vi "GetMethods.vi"(0 "ClassReaderNative in":refnum<class "ClassReaderNative.lvclass">, 5 "error in (no error)":errorcluster) -> (14 "ClassReaderNative out":refnum<class "ClassReaderNative.lvclass">, 15 "Methods":T1[](array[typedef]), 16 "Constructor/CreateIndex":i32, 19 "error out":errorcluster)   [LabVIEW 2014, in "ClassReaderNative.lvclass"]
uses:
  <resource>/Framework/Providers/Open_GDS/ClassProviders/Provider_LvNativeClass/ClassReaderNative_class/ClassReaderNative.lvclass
  <resource>/Framework/Providers/Open_GDS/ClassProviders/Provider_BaseClassInterface/Types/ClassTypes_MethodType.ctl
  <resource>/Framework/Providers/Open_GDS/ClassProviders/Provider_LvNativeClass/ClassReaderNative_class/ClassReaderNative.lvclass/ClassReaderNative.ctl
  <resource>/Framework/Providers/Open_GDS/ClassProviders/Provider_BaseClassInterface/ClassReader_class/ClassReader.lvclass
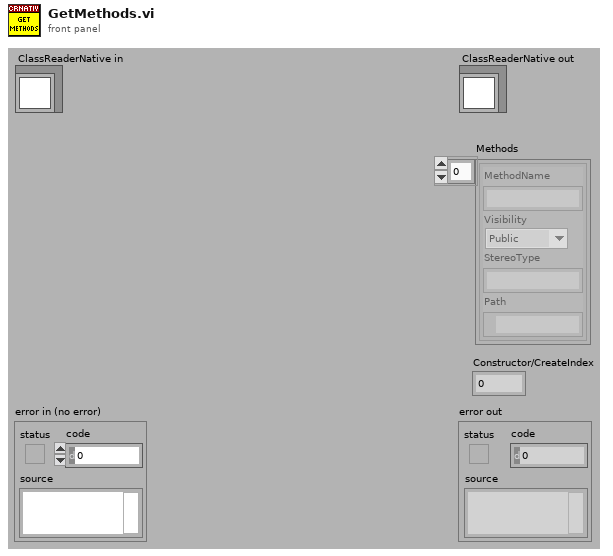
[diagram p1: front panel]
types:
  T1 = typedef "ClassTypes_MethodType.ctl" = cluster{"MethodName":string, "Visibility":enum16{"Public", "Private", "Protected"}, "StereoType":string, "Path":path}
  T2 = enum32{"invalid VI type", "Standard VI", "Control VI", "Global VI", "Polymorphic VI", "Configuration VI", "SubSystem", "Facade VI", "Method VI", "Statechart Diagram VI"}
  T3 = enum32{"invalid scope", "public", "private", "protected", "community"}
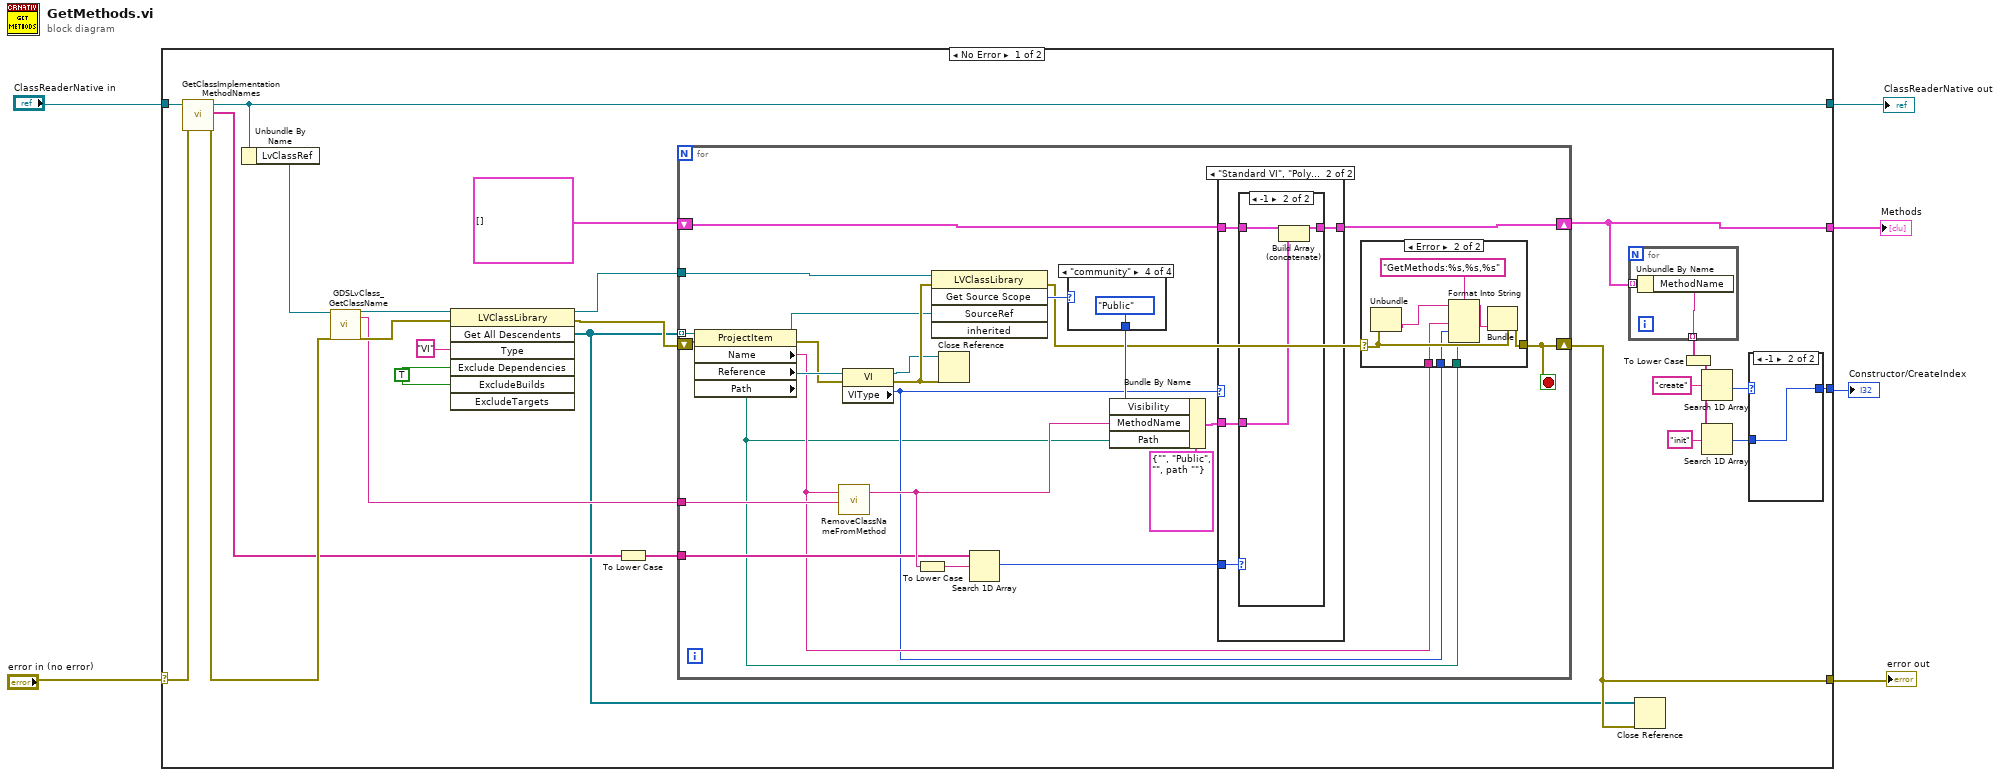
[diagram p0: block diagram]
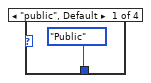
[diagram p6: hidden frame]
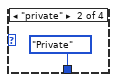
[diagram p7: hidden frame]
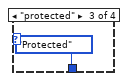
[diagram p8: hidden frame]
diagram:
  n1 = case shown="No Error" "error in (no error)" {
    selector: "error in (no error)" -> [w13 w82]
    tunnel: "ClassReaderNative in" -> [w15 w83]
    tunnel: [w14 w83] -> w4
    tunnel: [w23 _] -> w3
    tunnel: [w8 w82] -> w2
    tunnel: [w17 _] -> w1
    frame No Error {
      w9 = TRUE ("ExcludeDependencies")
      n2 = call-dynamic "GetClassImplementationMethodNames.vi"("error in (no error)"=w13, "ClassReaderNative in"=w15) -> ("error out"=w12:errorcluster, "ImplementationMethodNames"=w11:string[], "ClassReaderNative out"=w14:refnum<class "ClassReaderNative.lvclass">)  [unwired: 7 in]
      n3 = Unbundle By Name(w14) -> ("LvClassRef"=w24:refnum<vi>)
      n4 = call <resource>:"GDSLvClass_GetClassName.vi"("ViRef/Path,LvClassRef/Path"=w24, "error in (no error)"=w12) -> ("ClassRef"=w27:refnum<vi>, "ClassName(without .lvclass)"=w25:string, "error out"=w26:errorcluster)  [unwired: 15 in]
      n5 = invoke class="LVClassLibrary" method="Get All Descendents"(reference=w27, error in=w26, "Type"="VI", "Exclude Dependencies"=w9, "ExcludeBuilds"=w9) -> (reference out=w30:refnum<vi>, error out=w29:errorcluster, "All Descendents"=w7:refnum<vi>[])  [unwired: 2 in, 4 out]
      n6 = To Lower Case(string=w11) -> (all lower case string=w10:string[])
      n7 = for {
        tunnel: w7 -> [w59] mode=indexing
        tunnel: w30 -> [w58]
        shift-right: [w39] -> w8
        shift-left: w29 -> [w56]
        shift-right: [w53] -> w23
        shift-left: T1[] [] ("Methods") -> [w54]
        tunnel: w25 -> [w46]
        tunnel: w10 -> [w43]
        stop <- w39 stop-if-true
        n8 = property class="ProjectItem"(reference=w59, error in=w56) -> (reference out=w47:refnum<vi>, error out=w50:errorcluster, "Name"=w38:string, "Reference"=w55:refnum<vi>, "Path"=w36:path)
        n9 = call <resource>:"RemoveClassNameFromMethod.vi"("MethodVINameIn"=w38, "ClassName"=w46) -> ("MethodVINameOut"=w44:string)  [unwired: 17 in]
        n10 = property class="VI"(reference=w55, error in=w50) -> (reference out=w48:refnum<vi>, error out=w49:errorcluster, "VIType"=w37:T2)
        n11 = To Lower Case(string=w44) -> (all lower case string=w42:string)
        n12 = invoke class="LVClassLibrary" method="Get Source Scope"(reference=w58, error in=w49, "SourceRef"=w47) -> (error out=w40:errorcluster, "GetSourceScope"=w57:T3)  [unwired: 2 in, 3 out]
        n13 = Close Reference(reference=w48, error in (no error)=w49) -> ()  [unwired: 1 out]
        n14 = Search 1D Array(1D array=w43, element=w42) -> (index of element=w45:i32)  [unwired: 1 in]
        n15 = case shown="\"community\"" w57 {
          tunnel: [enum16{"Public", "Private", "Protected"}."Public" ("Visibility") enum16{"Public", "Private", "Protected"}."Private" ("Visibility") enum16{"Public", "Private", "Protected"}."Protected" ("Visibility") enum16{"Public", "Private", "Protected"}."Public" ("Visibility")] -> w41
          frame "public", Default {
          }
          frame "private" {
          }
          frame "protected" {
          }
          frame "community" {
          }
        }
        n16 = Bundle By Name(cluster=T1 {"MethodName"="", "Visibility"=enum."Public", "StereoType"="", "Path"=path ""} ("Method"), "Visibility"=w41, "MethodName"=w44, "Path"=w36) -> (w51:T1)
        n17 = case shown="\"Standard VI\", \"Polymorphic VI\", \"Facade VI\", \"Method VI\"" w37 {
          tunnel: w54 -> [w69 w73]
          tunnel: [w69 w72] -> w53
          tunnel: w51 -> [_ w71]
          tunnel: w45 -> [_ w70]
          frame Default {
          }
          frame "Standard VI", "Polymorphic VI", "Facade VI", "Method VI" {
            n18 = case shown="-1" w70 {
              tunnel: w73 -> [w74 w77]
              tunnel: [w74 w76] -> w72
              tunnel: w71 -> [_ w75]
              frame 0, Default {
              }
              frame -1 {
                n19 = Build Array (concatenate)(w77, w75) -> (w76:T1[])
              }
            }
          }
        }
        n20 = case shown="Error" w40 {
          selector: w40 -> [w60 w68]
          tunnel: [w60 w67] -> w39
          tunnel: w38 -> [_ w63]
          tunnel: w37 -> [_ w62]
          tunnel: w36 -> [_ w61]
          frame No Error {
          }
          frame Error {
            n21 = Unbundle(w68) -> ("source"=w66:string)  [unwired: 2 out]
            n22 = Format Into String(format string="GetMethods:%s,%s,%s", initial string=w66, w63, w62, w61) -> (resulting string=w65:string)  [unwired: 1 in, 1 out]
            n23 = Bundle(cluster=w68, "source"=w65) -> (w67:errorcluster)  [unwired: 2 in]
          }
        }
      }
      n24 = for {
        tunnel: w23 -> [w35] mode=indexing
        tunnel: [w34] -> w22 mode=indexing
        n25 = Unbundle By Name(w35) -> ("MethodName"=w34:string)
      }
      n26 = Close Reference(reference=w7, error in (no error)=w8) -> ()  [unwired: 1 out]
      n27 = To Lower Case(string=w22) -> (all lower case string=w20:string[])
      n28 = Search 1D Array(1D array=w20, element="create") -> (index of element=w18:i32)  [unwired: 1 in]
      n29 = Search 1D Array(1D array=w20, element="init") -> (index of element=w16:i32)  [unwired: 1 in]
      n30 = case shown="-1" w18 {
        selector: w18 -> [w32 _]
        tunnel: [w32 w33] -> w17
        tunnel: w16 -> [_ w33]
        frame Default {
        }
        frame -1 {
        }
      }
    }
    frame Error {
    }
  }
  "ClassReaderNative out" <- w4
  "Methods" <- w3
  "error out" <- w2
  "Constructor/CreateIndex" <- w1
